vi "Add Custom Device.vi"(8 "error in":errorcluster, 10 "name":string="Ballard ARINC 429", 11 "target in":refnum<k24>) -> (0 "error out":errorcluster, 2 "Ballard ARINC 429 custom device":T1 format="%.0x", 3 "target out":refnum<k24>)   [LabVIEW 2020, in "Ballard ARINC 429 Scripting.lvlib"]
doc: "Adds the Ballard ARINC 429 custom device to the system definition. Required sections for <b>Configuration Files</b>, <b>Incoming Ports</b>, <b>Outgoing Ports</b>, and <b>Status</b> are added within the custom device."
uses:
  Ballard ARINC 429 Scripting.lvlib
  NationalInstruments.VeriStand.SystemDefinitionAPI
  Constants.vi
  <vilib>/NI VeriStand/Custom Device Tools/Custom Device Utility Library/Custom Device Utility Library.lvlib
  <vilib>/NI VeriStand/Custom Device API/Custom Device Item Ref.ctl
  <vilib>/NI VeriStand/Custom Device API/Custom Device API.lvlib
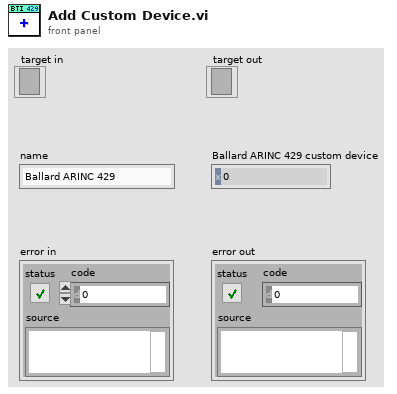
[diagram p1: front panel]
types:
  T1 = typedef "Custom Device API.lvlib/Custom Device Item Ref.ctl" = u64
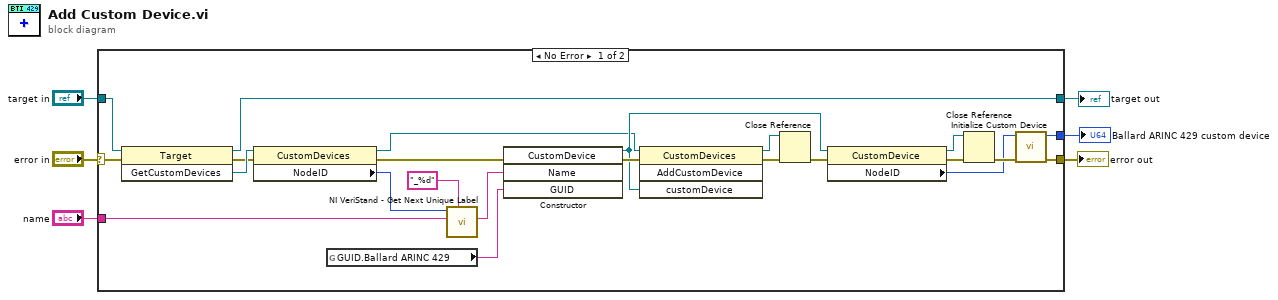
[diagram p0: block diagram]
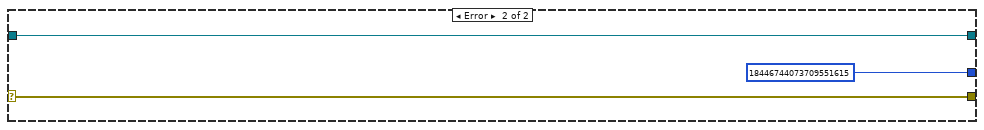
[diagram p2: hidden frame]
diagram:
  n1 = case shown="No Error" "error in" {
    selector: "error in" -> [w28 w32]
    tunnel: "target in" -> [w29 w31]
    tunnel: [w8 w32] -> w4
    tunnel: "name" -> [w16 _]
    tunnel: [w7 T1 18446744073709551615 ("Custom device Ref out")] -> w2
    tunnel: [w20 w31] -> w1
    frame No Error {
      n2 = invoke class="Target" method="GetCustomDevices"(reference=w29, error in=w28) -> (reference out=w20:refnum<k24>, error out=w13:errorcluster, "GetCustomDevices"=w18:refnum<k24>)  [unwired: 1 in]
      n3 = property class="CustomDevices"(reference=w18, error in=w13) -> (reference out=w11:refnum<k24>, error out=w12:errorcluster, "NodeID"=w17:u64)
      n4 = global read "Constants.vi" "GUID.Ballard ARINC 429"() -> (w19:string)
      n5 = call <vilib>:"NI VeriStand - Get Next Unique Label.vi"("format string"="_%d", "Label"=w16, "Parent Ref in"=w17) -> ("Label out"=w14:string)  [unwired: 5 in, 3 out]
      n6 = constructor class="CustomDevice"(error in=w12, "Name"=w14, "GUID"=w19) -> (reference out=w24:refnum<k24>, error out=w27:errorcluster)  [unwired: 2 in, 3 out]
      n7 = invoke class="CustomDevices" method="AddCustomDevice"(reference=w11, error in=w27, "customDevice"=w24) -> (reference out=w21:refnum<k24>, error out=w23:errorcluster)  [unwired: 1 in, 2 out]
      n8 = Close Reference(reference=w21, error in (no error)=w23) -> (error out=w22:errorcluster)
      n9 = property class="CustomDevice"(reference=w24, error in=w22) -> (reference out=w26:refnum<k24>, error out=w25:errorcluster, "NodeID"=w9:u64)
      n10 = Close Reference(reference=w26, error in (no error)=w25) -> (error out=w10:errorcluster)
      n11 = call "Initialize Custom Device.vi"("error in"=w10, "Ballard ARINC 429 ref"=w9) -> ("error out"=w8:errorcluster, "Ballard ARINC 429 ref out"=w7:T1)  [unwired: 8 in]
    }
    frame Error {
    }
  }
  "error out" <- w4
  "Ballard ARINC 429 custom device" <- w2
  "target out" <- w1
